vi "Reset Other Rs.vi"(8 "error in (no error)":errorcluster, 11 "IVI Refnum in":refnum<k15>) -> (0 "error out":errorcluster, 3 "IVI Refnum out":refnum<k15>)   [LabVIEW 2018]
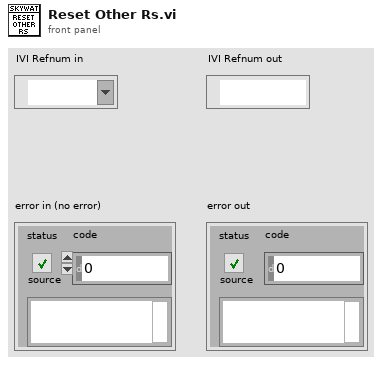
[diagram p1: front panel]
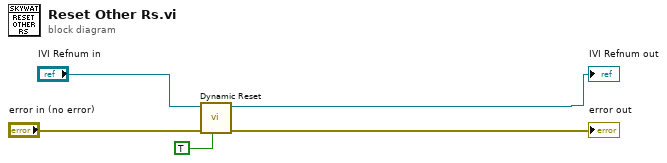
[diagram p0: block diagram]
diagram:
  n1 = call "Dynamic Reset.vi"("Reset all others?"=TRUE ("reset?"), "error in (no error)"="error in (no error)", "instrument handle"="IVI Refnum in") -> ("error out"=→"error out":errorcluster, "instrument handle out"=→"IVI Refnum out":refnum<k15>)  [unwired: 2 in, 5 out]
